vi "Load Data.vi"(8 "error in (no error)":errorcluster, 10 "Data":cluster{"Numeric":i32}, 11 "CutomOOB_Rx in":refnum<class "CIFTCustomOOB_Rx.lvclass">) -> (0 "error out":errorcluster, 3 "CutomOOB_Rx out":refnum<class "CIFTCustomOOB_Rx.lvclass">)   [LabVIEW 2021, in "CIFTCustomOOB_Rx.lvclass"]
uses:
  CIFTCustomOOB_Rx.lvclass
  D:/dev/CIF-LVCore/src/CIFUtilities/CIFOutOfBand/CIFOutOfBand.lvclass
  CIFUtilities/CIFOutOfBand/CIFOutOfBand.lvclass/CIFOutOfBand.ctl
  Typedef/Payload.ctl
  CIFUtilities/CIFOutOfBand/CIFOutOfBand.lvclass
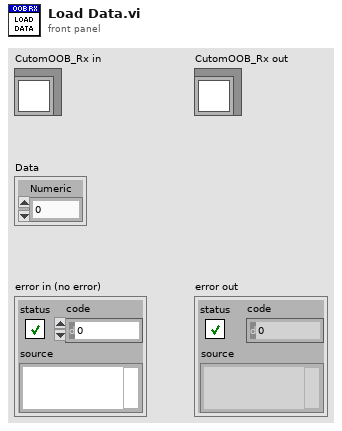
[diagram p1: front panel]
types:
  T1 = typedef "CIFTCustomOOB_Rx.lvclass/Payload.ctl" = cluster{"Data":cluster{"Numeric":i32}}
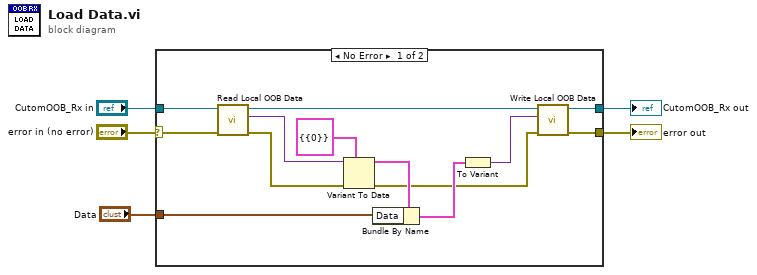
[diagram p0: block diagram]
diagram:
  n1 = case shown="No Error" "error in (no error)" {
    selector: "error in (no error)" -> [w11 w20]
    tunnel: [w18 w20] -> w5
    tunnel: [w17 w19] -> w4
    tunnel: "CutomOOB_Rx in" -> [w14 w19]
    tunnel: "Data" -> [w6 _]
    frame No Error {
      n2 = call "Read Local OOB Data.vi"("error in"=w11, "OOB in"=w14) -> ("error out"=w8:errorcluster, "Local OOB Data"=w12:variant, "OOB out"=w13:refnum<class "CIFTCustomOOB_Rx.lvclass">)  [unwired: 7 in]
      n3 = Variant To Data(error in=w8, type=T1 {"Data"={"Numeric"=0}} ("Template Payload"), Variant=w12) -> (data=w9:T1, error out=w7:errorcluster)
      n4 = Bundle By Name(cluster=w9, "Data"=w6) -> (w16:T1)
      n5 = To Variant(anything=w16) -> (Variant=w15:variant)
      n6 = call "Write Local OOB Data.vi"("error in"=w7, "Local OOB Data"=w15, "OOB in"=w13) -> ("error out"=w18:errorcluster, "OOB out"=w17:refnum<class "CIFTCustomOOB_Rx.lvclass">)  [unwired: 7 in]
    }
    frame Error {
    }
  }
  "error out" <- w5
  "CutomOOB_Rx out" <- w4
